vi "Post-Build Action.vi"(5 "Files Generated by Build":path[](array[path]), 6 "Top Level/Always Included VIs":path[](array[path]), 7 "Destination Path":path, 8 "error in (no error)":errorcluster, 9 "Target Name":string, 10 "Build Specification Name":string, 11 "Project Path":path) -> (0 "error out":errorcluster)   [LabVIEW 2020]
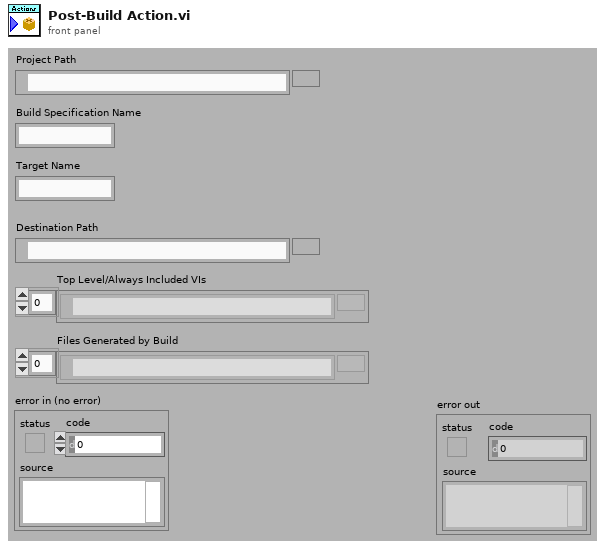
[diagram p1: front panel]
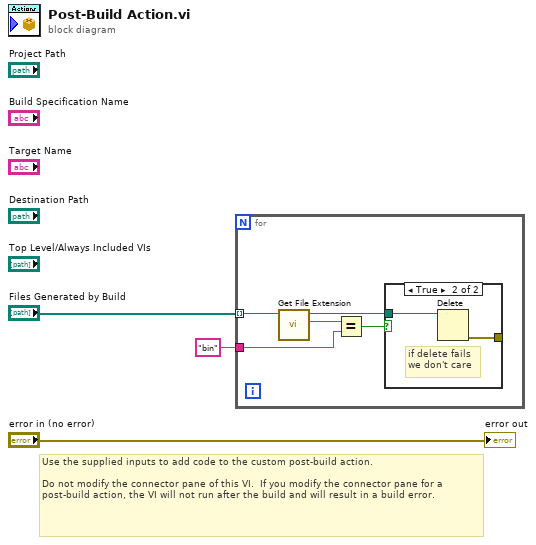
[diagram p0: block diagram]
diagram:
  # "Use the supplied inputs to add code to the custom post-build action.\n\nDo not modify the connector pane of this VI.  If you modify the connector pane for a post-build action, the VI will not run after the build and will result in a build error."
  n1 = for {
    tunnel: "Files Generated by Build" -> [w8] mode=indexing
    tunnel: "bin" -> [w6]
    n2 = call <vilib>:"Get File Extension.vi"("file"=w8) -> ("lowercase file extension"=w7:string, "dup file"=w4:path)  [unwired: 6 in, 3 out]
    n3 = Equal?(x=w7, y=w6) -> (x = y?=w5:bool)
    n4 = case shown="True" w5 {
      tunnel: w4 -> [_ w10]
      tunnel: [_ w9] -> _
      frame False {
      }
      frame True {
        # "if delete fails\nwe don't care"
        n5 = Delete(path (use dialog)=w10) -> (error out=w9:errorcluster)  [unwired: 4 in, 2 out]
      }
    }
  }
  "error out" <- "error in (no error)"
